vi "Software Update HCC Determine LV Software Version.vi"(8 "Error In":errorcluster, 9 "Search Expression in":string, 10 "Filenames Input":string[](array[string]), 11 "Input Path":path) -> (0 "Error Out":errorcluster, 3 "Output Path":path[](array[path]), 4 "Software Version":string)   [LabVIEW 2016]
panel:
  in  "Strip Archive Folder?":enum16{"Yes", "No"}(ring)
  out "Path of Checked Version":path
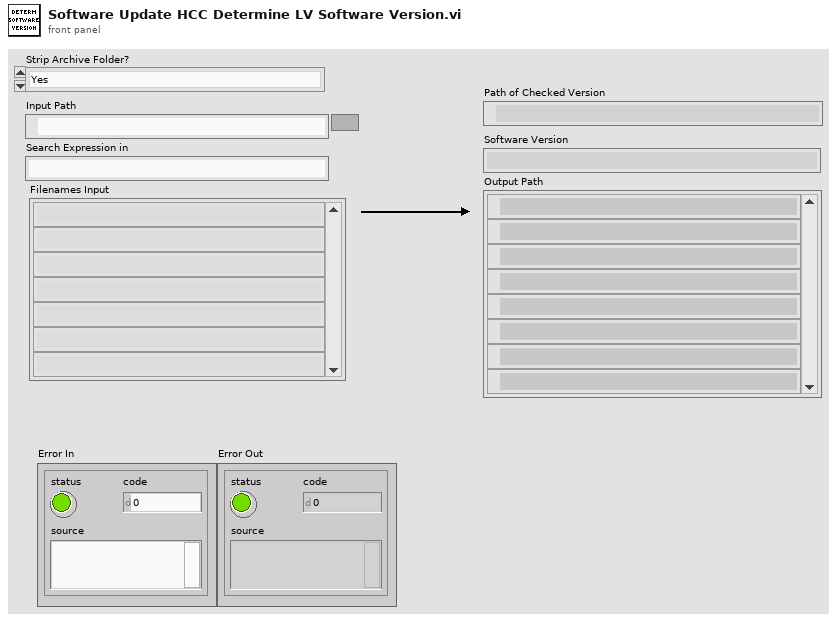
[diagram p1: front panel]
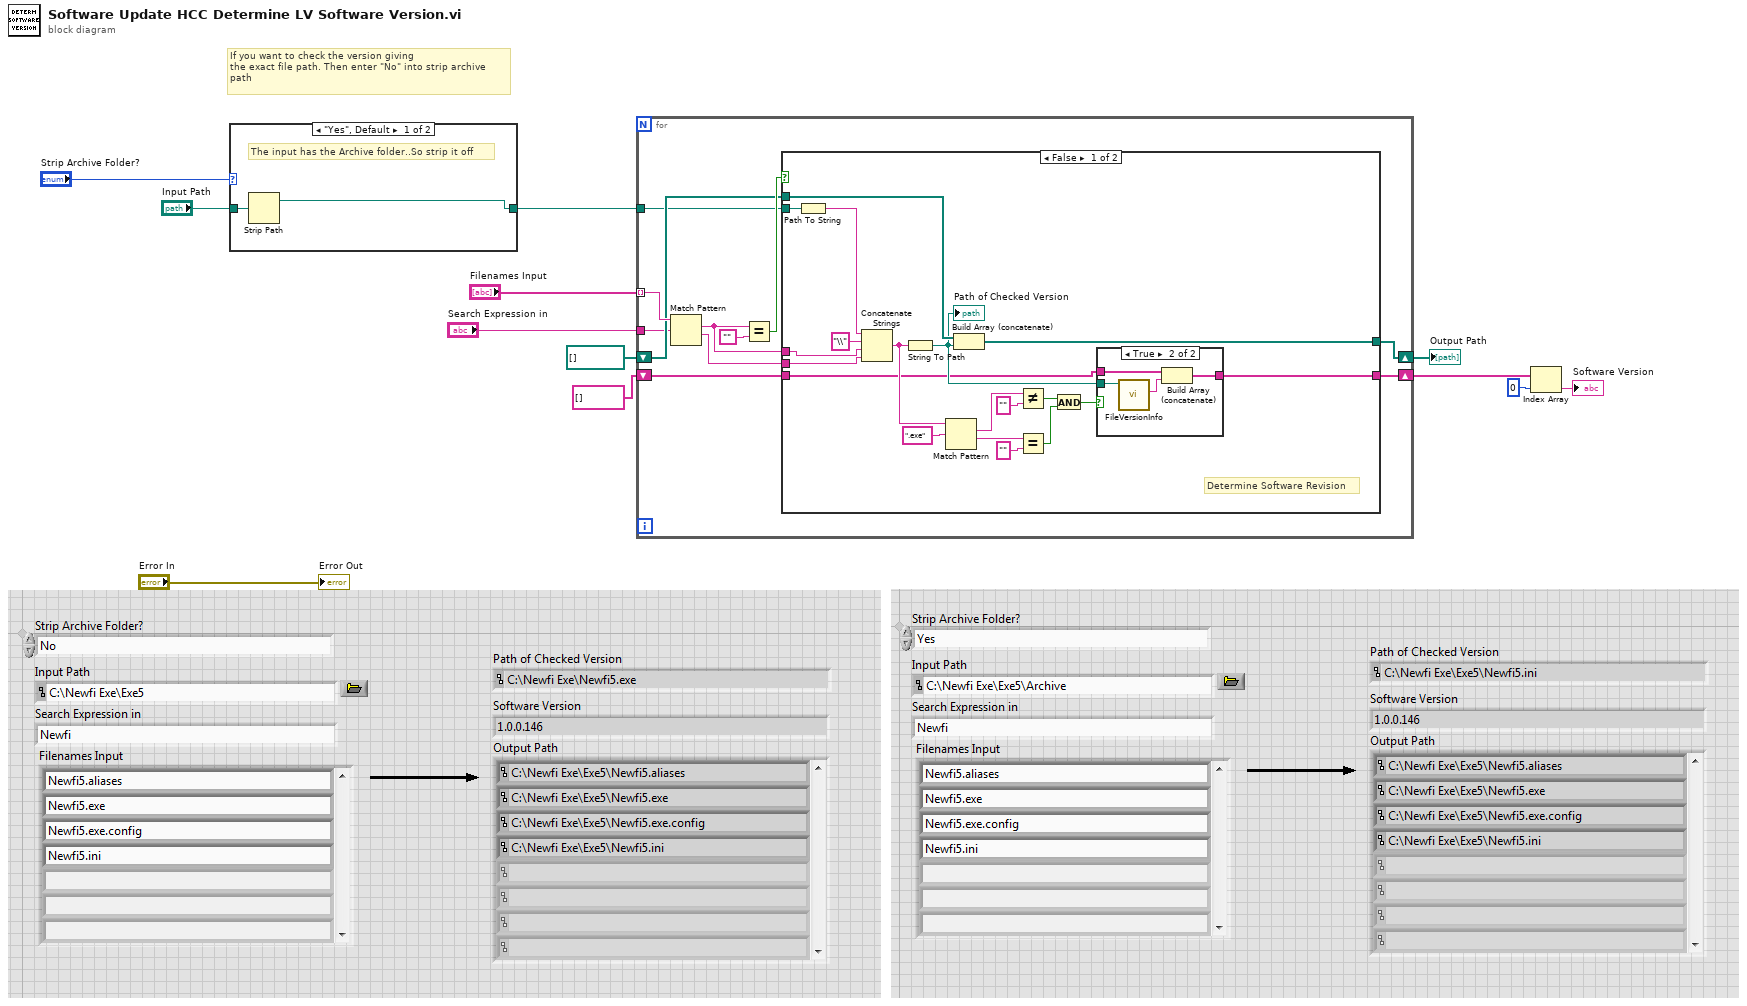
[diagram p0: block diagram]
diagram:
  # "If you want to check the version giving \nthe exact file path. Then enter \"No\" into strip archive \npath"
  n1 = case shown="\"Yes\", Default" "Strip Archive Folder?" {
    tunnel: "Input Path" -> [w14 w15]
    tunnel: [w13 w15] -> w5
    frame "Yes", Default {
      # "The input has the Archive folder..So strip it off"
      n2 = Strip Path(path=w14) -> (stripped path=w13:path)  [unwired: 1 out]
    }
    frame "No" {
    }
  }
  n3 = for {
    tunnel: "Filenames Input" -> [w26] mode=indexing
    shift-right: [w22] -> w12
    shift-left: path[] [] -> [w23]
    tunnel: "Search Expression in" -> [w19]
    tunnel: w5 -> [w18]
    shift-right: [w16] -> w7
    shift-left: string[] [] -> [w17]
    n4 = Match Pattern(string=w26, regular expression=w19) -> (match substring=w21:string, after substring=w20:string)  [unwired: 1 in, 2 out]
    n5 = Equal?(x=w21, y="") -> (x = y?=w24:bool)
    n6 = case shown="False" w24 {
      tunnel: w23 -> [w45 w52]
      tunnel: [w44 w52] -> w22
      tunnel: w21 -> [w43 _]
      tunnel: w20 -> [w42 _]
      tunnel: w18 -> [w41 _]
      tunnel: w17 -> [w28 w51]
      tunnel: [w27 w51] -> w16
      frame False {
        # "Determine Software Revision"
        n7 = Path To String(path=w41) -> (string=w40:string)
        n8 = Concatenate Strings(w40, "\\" ("string"), w43, w42) -> (w38:string)
        n9 = String To Path(string=w38) -> (path=w29:path)
        "Path of Checked Version" <- w29
        n10 = Match Pattern(string=w38, regular expression=".exe") -> (match substring=w34:string, after substring=w36:string)  [unwired: 1 in, 2 out]
        n11 = Build Array (concatenate)(w45, w29) -> (w44:path[])
        n12 = Not Equal?(x=w34, y="") -> (x != y?=w32:bool)
        n13 = Equal?(x=w36, y="") -> (x = y?=w31:bool)
        n14 = And(x=w32, y=w31) -> (x .and. y?=w30:bool)
        n15 = case shown="True" w30 {
          tunnel: w29 -> [_ w50]
          tunnel: w28 -> [w46 w49]
          tunnel: [w46 w47] -> w27
          frame False {
          }
          frame True {
            n16 = call <vilib>:"FileVersionInfo.vi"("Application Path in"=w50) -> ("File Version Info"=w48:string)  [unwired: 7 in, 3 out]
            n17 = Build Array (concatenate)(w49, w48) -> (w47:string[])
          }
        }
      }
      frame True {
      }
    }
  }
  "Output Path" <- w12
  n18 = Index Array(array=w7, index=0) -> (element=→"Software Version":string)
  "Error Out" <- "Error In"
